vi "MFLI Initiate module.vi"(10 "Mode":T1, 11 "ACQ  status in":T2 {"ModuleHandles"."ModHandle" format="0x%08x"; "ModuleHandles"."Conn" format="0x%08x"; "Lock-in Handle"."Handle" format="0x%08x"; "Lock-in Handle"."Conn" format="0x%08x"}) -> (3 "ACQ  status out":T2 {"ModuleHandles"."ModHandle" format="0x%08x"; "ModuleHandles"."Conn" format="0x%08x"; "Lock-in Handle"."Handle" format="0x%08x"; "Lock-in Handle"."Conn" format="0x%08x"})   [LabVIEW 2017]
uses:
  <instrlib>/Zurich Instruments LabOne/Public/Modules/ziTypeModEnum.ctl
  <instrlib>/Zurich Instruments LabOne/Zurich Instruments LabOne.lvlib
  <instrlib>/Zurich Instruments LabOne/Public/Modules/ziModSetValueDoubleArray.vi
  Lock-in module.lvlib
  <instrlib>/Zurich Instruments LabOne/Public/Modules/ziModSetValueBinary.vi
  <instrlib>/Zurich Instruments LabOne/Public/Configure/ziSetValueDoubleArray.vi
  <instrlib>/Zurich Instruments LabOne/Public/ziTypeHandle.ctl
  <instrlib>/Zurich Instruments LabOne/Public/Modules/ziTypeModHandle.ctl
  ctl/ACQ info.ctl
  ctl/ACQ status.ctl
  ctl/Mode.ctl
panel:
  out "Selected Device":string
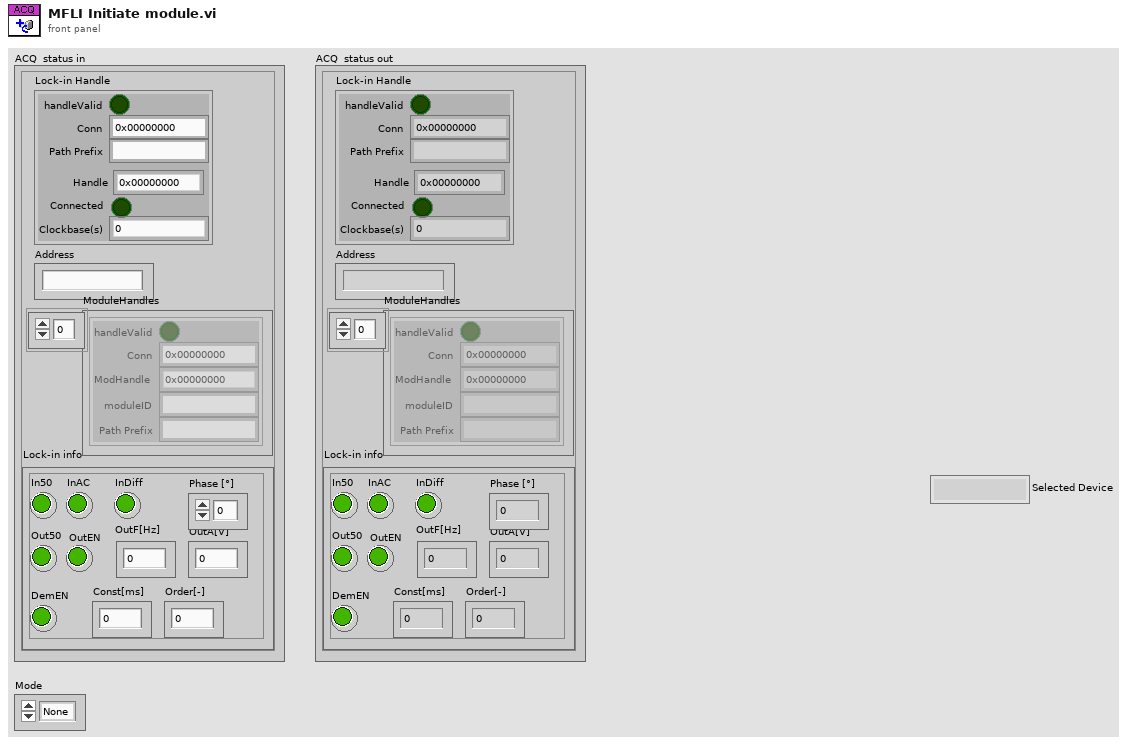
[diagram p1: front panel]
types:
  T1 = typedef "Lock-in module.lvlib/Mode.ctl" = enum16{"None", "Point", "Scope", "Both", "DAQ"}
  T2 = typedef "Lock-in module.lvlib/ACQ status.ctl" = cluster{"Lock-in Handle":T3, "Address":string, "ModuleHandles":T4[], "Lock-in info":T5}
  T3 = typedef "Zurich Instruments LabOne.lvlib/ziTypeHandle.ctl" = cluster{"handleValid":bool, "Conn":u64, "Path Prefix":string, "Handle":u64, "Connected":bool, "Clockbase(s)":dbl}
  T4 = typedef "Zurich Instruments LabOne.lvlib/ziTypeModHandle.ctl" = cluster{"handleValid":bool, "Conn":u64, "ModHandle":u64, "moduleID":string, "Path Prefix":string}
  T5 = typedef "Lock-in module.lvlib/ACQ info.ctl" = cluster{"In50":bool, "InAC":bool, "InDiff":bool, "Out50":bool, "OutEN":bool, "OutF[Hz]":dbl, "OutA[V]":dbl, "DemEN":bool, "Const[ms]":dbl, "Order[-]":i32, "Phase [°]":dbl}
  T6 = typedef "Zurich Instruments LabOne.lvlib/ziTypeModEnum.ctl" = u16
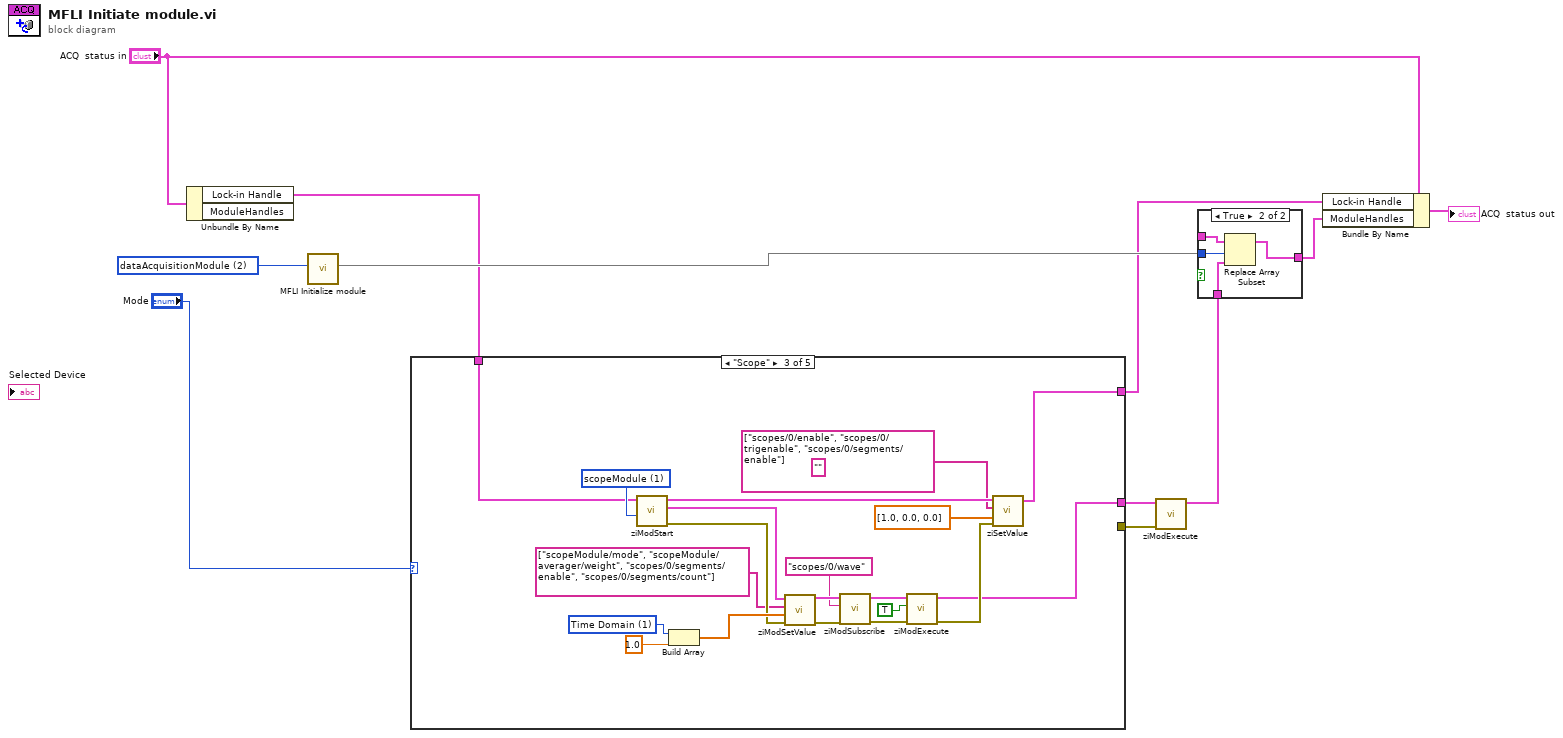
[diagram p0: block diagram]
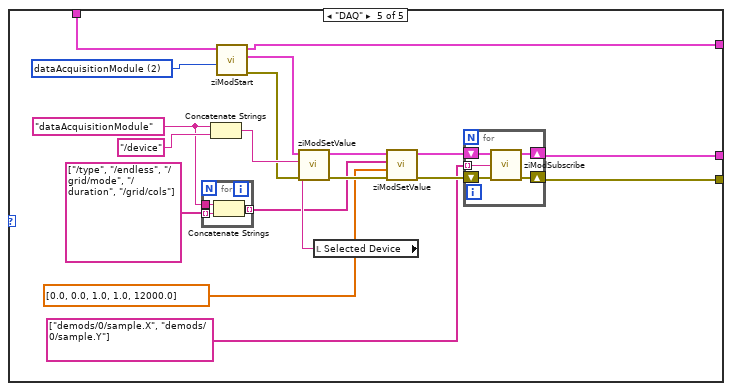
[diagram p5: hidden frame]
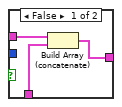
[diagram p6: hidden frame]
diagram:
  w1 = T6 2 items=["sweep", "scopeModule", "dataAcquisitionModule", "pidAdvisor", "awgModule", "impedanceModule", "multiDeviceSyncModule", "zoomFFT", "trigger", "deviceSettings", "record"] ("module Id")
  n1 = Unbundle By Name("ACQ  status in") -> ("Lock-in Handle"=w3:T3)  [unwired: 1 out]
  n2 = call "MFLI Initialize module.vi"("module Id"=w1) -> (2:w5)  [unwired: 8 in, 2 out]
  n3 = case shown="\"Scope\"" "Mode" {
    tunnel: [_ _ _ _ w53] -> w9
    tunnel: [_ _ w15 _ w52] -> w8
    tunnel: w3 -> [w12 w13 w14 w34 w39]
    tunnel: [w12 w13 w16 w34 w37] -> w2
    frame "None", Default {
    }
    frame "Point" {
    }
    frame "Scope" {
      w22 = u16 1 items=["Time Domain"=1, "Freq Domain FFT"=3] ("mode")
      w19 = T6 1 items=["sweep", "scopeModule", "dataAcquisitionModule", "pidAdvisor", "awgModule", "impedanceModule", "multiDeviceSyncModule", "zoomFFT", "trigger", "deviceSettings", "record"] ("module Id")
      (unwired) ""
      n4 = call <instrlib>:"ziModStart.vi"("module Id"=w19, "Handle In"=w14) -> ("Error Out"=w31:errorcluster, "ModHandle Out"=w30:T4, "Handle Out"=w32:T3)  [unwired: 7 in]
      n5 = Build Array(w22, 1.0 ("averagerweight")) -> (w33:dbl[])
      n6 = call-poly <instrlib>:"ziModSetValue.vi"("Error In"=w31, "Values"=w33, "Paths"=string[] ["scopeModule/mode", "scopeModule/averager/weight", "scopes/0/segments/enable", "scopes/0/segments/count"], "ModHandle In"=w30) -> ("Error Out"=w26:errorcluster, "ModHandle Out"=w27:T4)  [unwired: 6 in]
      n7 = call <instrlib>:"ziModSubscribe.vi"("Error In"=w26, "Path"="scopes/0/wave", "ModHandle In"=w27) -> ("Error Out"=w28:errorcluster, "ModHandle Out"=w29:T4)  [unwired: 6 in]
      n8 = call <instrlib>:"ziModExecute.vi"("Error In"=w28, "Modal (F)"=TRUE ("Modal"), "ziModHandle In"=w29) -> ("Error Out"=w25:errorcluster, "ziModHandle Out"=w15:T4)  [unwired: 5 in, 1 out]
      n9 = call-poly <instrlib>:"ziSetValue.vi"("Error In"=w25, "Values"=dbl[] [1.0, 0.0, 0.0] ("Value"), "Paths"=string[] ["scopes/0/enable", "scopes/0/trigenable", "scopes/0/segments/enable"], "Handle In"=w32) -> ("Handle Out"=w16:T3)  [unwired: 1 in, 1 out]
    }
    frame "Both" {
    }
    frame "DAQ" {
      w36 = T6 2 items=["sweep", "scopeModule", "dataAcquisitionModule", "pidAdvisor", "awgModule", "impedanceModule", "multiDeviceSyncModule", "zoomFFT", "trigger", "deviceSettings", "record"] ("module Id")
      w41 = "dataAcquisitionModule"
      n10 = for {
        tunnel: string[] ["/type", "/endless", "/grid/mode", "/duration", "/grid/cols"] -> [w56] mode=indexing
        tunnel: w41 -> [w55]
        tunnel: [w54] -> w40 mode=indexing
        n11 = Concatenate Strings(w55, w56) -> (w54:string)
      }
      n12 = Concatenate Strings(w41, "/device") -> (w43:string)
      n13 = call <instrlib>:"ziModStart.vi"("module Id"=w36, "Handle In"=w39) -> ("Error Out"=w35:errorcluster, "ModHandle Out"=w38:T4, "Handle Out"=w37:T3)  [unwired: 7 in]
      n14 = local read "Selected Device"() -> (w45:string)
      n15 = call-poly <instrlib>:"ziModSetValue.vi"("Error In"=w35, "Data"=w45, "Path"=w43, "ModHandle In"=w38) -> ("Error Out"=w48:errorcluster, "ModHandle Out"=w47:T4)  [unwired: 6 in]
      n16 = call-poly <instrlib>:"ziModSetValue.vi"("Error In"=w48, "Values"=dbl[] [0.0, 0.0, 1.0, 1.0, 12000.0], "Paths"=w40, "ModHandle In"=w47) -> ("Error Out"=w50:errorcluster, "ModHandle Out"=w51:T4)  [unwired: 6 in]
      n17 = for {
        shift-right: [w61] -> w52
        shift-left: w51 -> [w58]
        tunnel: string[] ["demods/0/sample.X", "demods/0/sample.Y"] ("subscribe") -> [w60] mode=indexing
        shift-right: [w57] -> w53
        shift-left: w50 -> [w59]
        n18 = call <instrlib>:"ziModSubscribe.vi"("Error In"=w59, "Path"=w60, "ModHandle In"=w58) -> ("Error Out"=w57:errorcluster, "ModHandle Out"=w61:T4)  [unwired: 6 in]
      }
    }
  }
  n19 = call <instrlib>:"ziModExecute.vi"("Error In"=w9, "ziModHandle In"=w8) -> ("ziModHandle Out"=w6:T4)  [unwired: 6 in, 2 out]
  n20 = case shown="True" {
    selector: _ -> [_ _]
    tunnel: [w64 w65] -> w7
    tunnel: _ -> [w63 w68]
    tunnel: w6 -> [w62 w66]
    tunnel: w5 -> [_ w67]
    frame False {
      n21 = Build Array (concatenate)(w63, w62) -> (w64:T4[])
    }
    frame True {
      n22 = Replace Array Subset(array=w68, new element=w66, index=w67) -> (w65:T4[])
    }
  }
  n23 = Bundle By Name(cluster="ACQ  status in", "Lock-in Handle"=w2, "ModuleHandles"=w7) -> (→"ACQ  status out":T2)
